vi "Reconnect.vi"(8 "error in":errorcluster, 10 "Reconnect Parameters":T2={"IP Address"="", "JSON"="", "bytes to read (1024)"=1024, "timeout ms (5)"=5, "port (4222)"=4222}, 11 "nats connection in":T1={"connection ID"=refnum, "server INFO"="", "timeout ms"=5000, "verbose?"=FALSE, "server headers?"=FALSE, "client headers?"=FALSE}) -> (0 "error out":errorcluster, 2 "CONNECT processed?":bool, 3 "nats connection out":T1={"connection ID"=refnum, "server INFO"="", "timeout ms"=5000, "verbose?"=FALSE, "server headers?"=FALSE, "client headers?"=FALSE})   [LabVIEW 2020, in "NATS Client.lvlib" / "NATS Client.lvclass"]
uses:
  NATS Client.lvclass
  <vilib>/NATS/NATS Core/NATS Core.lvlib
  Reconnect Parameters.ctl
  <vilib>/NATS/NATS Core/Controls/nats connection.ctl
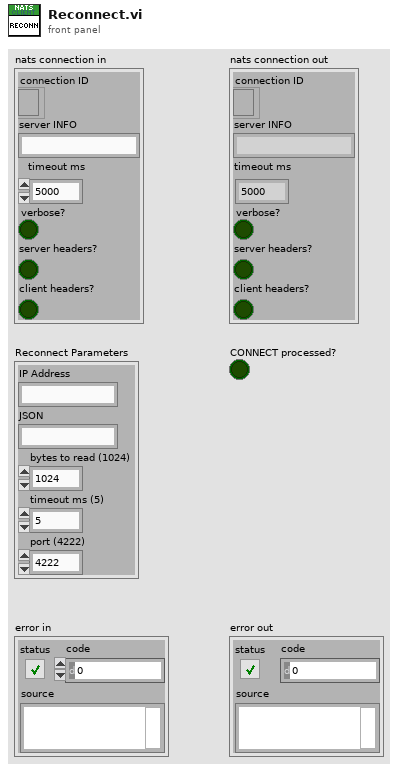
[diagram p1: front panel]
types:
  T1 = typedef "NATS Core.lvlib/nats connection.ctl" = cluster{"connection ID":refnum<k5>, "server INFO":string, "timeout ms":i32, "verbose?":bool, "server headers?":bool, "client headers?":bool}
  T2 = typedef "NATS Client.lvlib/NATS Client.lvclass/Reconnect Parameters.ctl" = cluster{"IP Address":string, "JSON":string, "bytes to read (1024)":i32, "timeout ms (5)":i32, "port (4222)":u16}
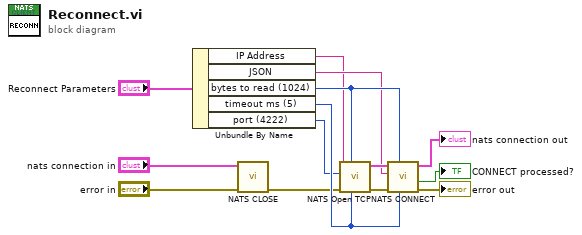
[diagram p0: block diagram]
diagram:
  n1 = Unbundle By Name("Reconnect Parameters") -> ("IP Address"=w3:string, "JSON"=w4:string, "bytes to read (1024)"=w7:i32, "timeout ms (5)"=w6:i32, "port (4222)"=w5:u16)
  n2 = call <vilib>:"NATS CLOSE.vi"("error in"="error in", "nats connection in"="nats connection in") -> ("error out"=w1:errorcluster)  [unwired: 9 in]
  n3 = call <vilib>:"NATS Open TCP.vi"("timeout ms (5000)"=w6, "bytes to read (1024)"=w7, "error in"=w1, "port (4222)"=w5, "address"=w3) -> ("error out"=w14:errorcluster, "nats connection"=w13:T1)  [unwired: 3 in, 2 out]
  n4 = call <vilib>:"NATS CONNECT.vi"("timeout ms (conn default)"=w6, "bytes to read (1024)"=w7, "error in"=w14, "JSON"=w4, "nats connection in"=w13) -> ("error out"=→"error out":errorcluster, "CONNECT processed?"=→"CONNECT processed?":bool, "nats connection out"=→"nats connection out":T1)  [unwired: 4 in]
